vi "LS330_DequLog.vi"(8 "error in":errorcluster, 11 "Queue in":refnum<queue>) -> (0 "error out":errorcluster, 1 "Status Out":cluster{T1, T1}, 2 "Time Stamp":timestamp, 3 "Queue out":refnum<queue>, 5 "Terminate?":bool, 6 "Status/Time  Out":T2)   [LabVIEW 2021]
uses:
  LS330_Status_Bundle.ctl
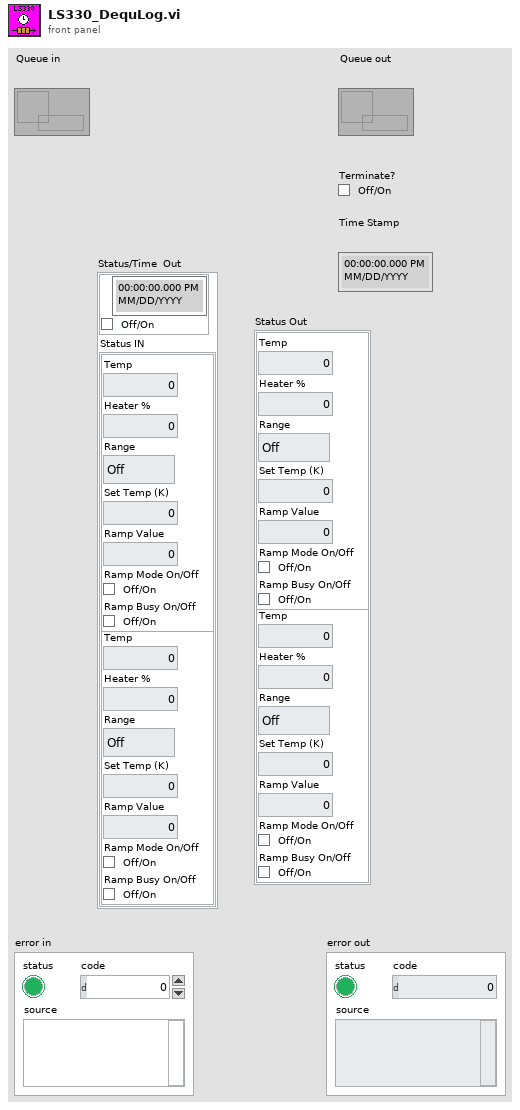
[diagram p1: front panel]
types:
  T1 = typedef "LS330_Status_Bundle.ctl" = cluster{"Temp":dbl, "Heater %":dbl, "Range":enum16{"Off", "Low", "Medium", "High"}, "Set Temp (K)":dbl, "Ramp Value":dbl, "Ramp Mode On/Off":bool, "Ramp Busy On/Off":bool}
  T2 = cluster{"Cluster":cluster{timestamp, "Checkbox":bool}, "Status IN":cluster{T1, T1}}
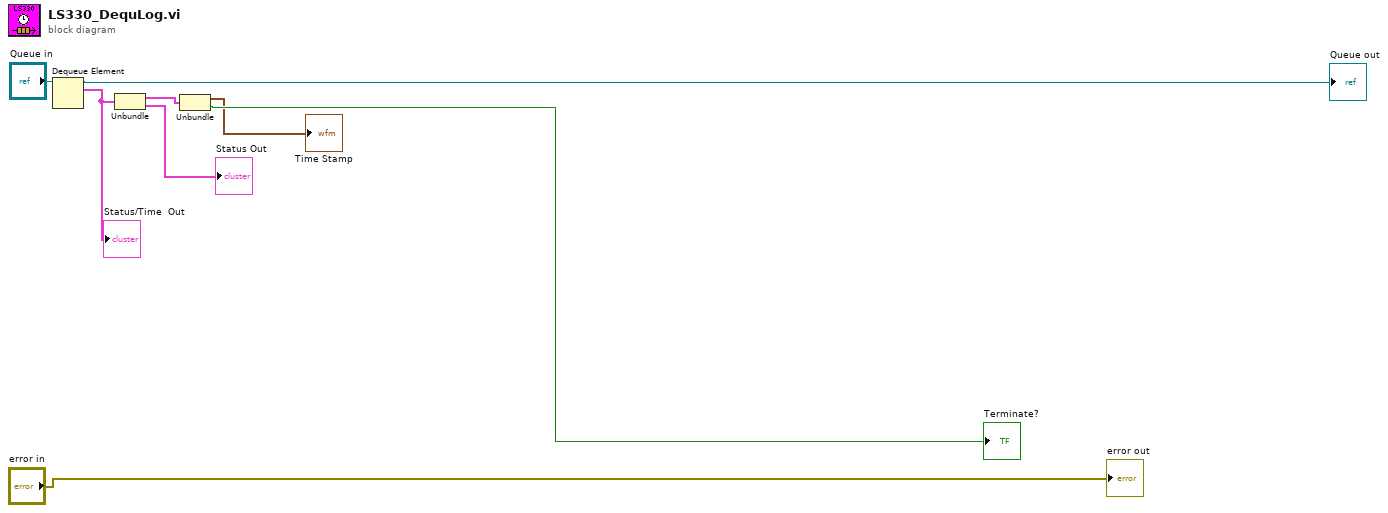
[diagram p0: block diagram]
diagram:
  n1 = Dequeue Element(queue="Queue in") -> (queue out=→"Queue out":refnum<queue>, element=w7:T2)  [unwired: 2 in, 2 out]
  "Status/Time  Out" <- w7
  n2 = Unbundle(w7) -> ("Cluster"=w4:cluster{timestamp, "Checkbox":bool}, "Status IN"=→"Status Out":cluster{T1, T1})
  n3 = Unbundle(w4) -> (→"Time Stamp":timestamp, "Checkbox"=→"Terminate?":bool)
  "error out" <- "error in"
